vi "Example.vi"() -> ()   [LabVIEW 2009]
panel:
  in  "Move To":dbl
  out "Position":dbl
  out "Closing Error":errorcluster
  out "Running Error":errorcluster
  in  "stop":bool
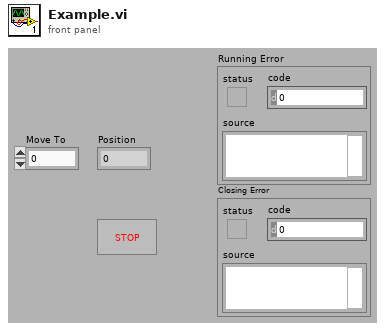
[diagram p1: front panel]
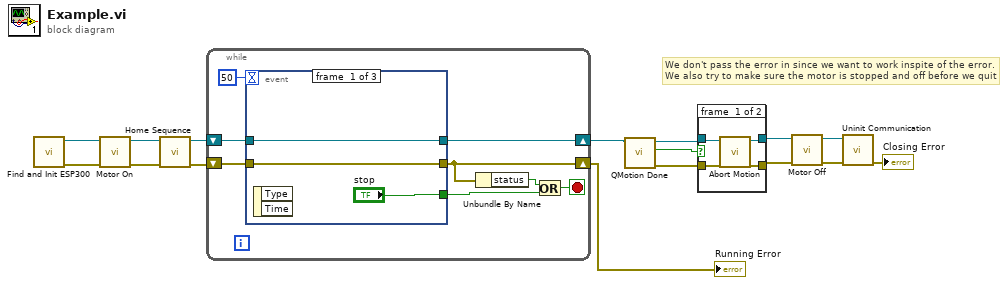
[diagram p0: block diagram]
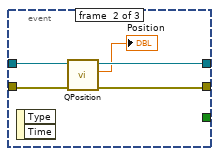
[diagram p3: hidden frame]
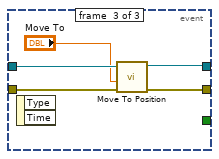
[diagram p4: hidden frame]
diagram:
  # "We don't pass the error in since we want to work inspite of the error.\nWe also try to make sure the motor is stopped and off before we quit"
  n1 = call "Find and Init ESP300.vi"() -> ("error out"=w15:errorcluster, "VISA resource name out"=w16:refnum<visa-resource-name>)  [unwired: 10 in]
  n2 = call "Motor On.vi"("error in (no error)"=w15, "VISA resource name in"=w16) -> ("error out"=w13:errorcluster, "VISA resource name out"=w14:refnum<visa-resource-name>)  [unwired: 8 in]
  n3 = call "Home Sequence.vi"("error out in (no error)"=w13, "VISA resource name"=w14) -> ("error out"=w12:errorcluster, "VISA resource name out"=w11:refnum<visa-resource-name>)  [unwired: 8 in]
  n4 = while {
    shift-right: [w20] -> w10
    shift-left: w12 -> [w22]
    shift-right: [w23] -> w8
    shift-left: w11 -> [w24]
    stop <- w18 stop-if-true
    n5 = event shown="[1] Timeout" {
      selector: _ -> [_ _ _]
      dyn-events: _ -> [_ _ _]
      timeout: 50 -> [_ _ _]
      tunnel: ["stop" _ _] -> w21
      tunnel: w24 -> [w26 w32 w37]
      tunnel: [w26 w29 w35] -> w23
      tunnel: w22 -> [w25 w31 w36]
      tunnel: [w25 w30 w34] -> w20
      event #0 {
        n6 = event-data() -> ()  [unwired: 1 in, 2 out]
      }
      event #1 {
        n7 = event-data() -> ()  [unwired: 1 in, 2 out]
        n8 = call "QPosition.vi"("error in (no error)"=w31, "VISA resource name in"=w32) -> ("error out"=w30:errorcluster, "Position"=→"Position":dbl, "VISA resource name out"=w29:refnum<visa-resource-name>)  [unwired: 7 in]
      }
      event #2 {
        n9 = event-data() -> ()  [unwired: 1 in, 2 out]
        n10 = call "Move To Position.vi"("error in (no error)"=w36, "Postion (Unit)"="Move To", "VISA resource name in"=w37) -> ("error out"=w34:errorcluster, "VISA resource name out"=w35:refnum<visa-resource-name>)  [unwired: 7 in]
      }
    }
    n11 = Unbundle By Name(w20) -> ("status"=w19:bool)
    n12 = Or(x=w19, y=w21) -> (x .or. y?=w18:bool)
  }
  "Running Error" <- w10
  n13 = call "QMotion Done.vi"("VISA resource name in"=w8) -> ("error out"=w5:errorcluster, "Motion Done?"=w7:bool, "VISA resource name out"=w6:refnum<visa-resource-name>)  [unwired: 8 in]
  n14 = case shown="False" w7 {
    tunnel: w6 -> [w41 w43]
    tunnel: w5 -> [w40 w42]
    tunnel: [w38 w43] -> w4
    tunnel: [w39 w42] -> w3
    frame #0 {
      n15 = call "Abort Motion.vi"("error in (no error)"=w40, "VISA resource name in"=w41) -> ("error out"=w39:errorcluster, "VISA resource name out"=w38:refnum<visa-resource-name>)  [unwired: 8 in]
    }
    frame #1 {
    }
  }
  n16 = call "Motor Off.vi"("error in (no error)"=w3, "VISA resource name in"=w4) -> ("error out"=w2:errorcluster, "VISA resource name out"=w1:refnum<visa-resource-name>)  [unwired: 8 in]
  n17 = call "Uninit Communication.vi"("error in (no error)"=w2, "VISA resource name in"=w1) -> ("error out"=→"Closing Error":errorcluster)  [unwired: 9 in]
